vi "mtg reader - get short file names.vi"(6 "rowsize":i32=6, 9 "session file selection":refnum<vi>, 10 "session files in":refnum<vi>, 11 "data (session)":path) -> (2 "session files out":refnum<vi>)   [LabVIEW 2025]
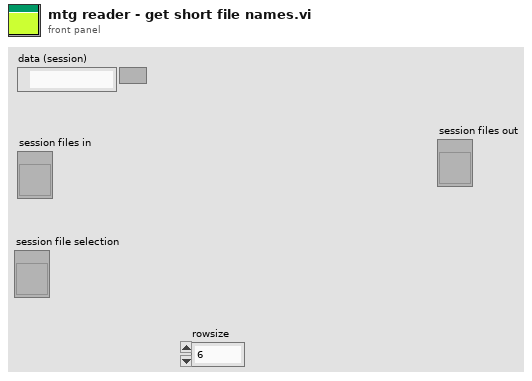
[diagram p1: front panel]
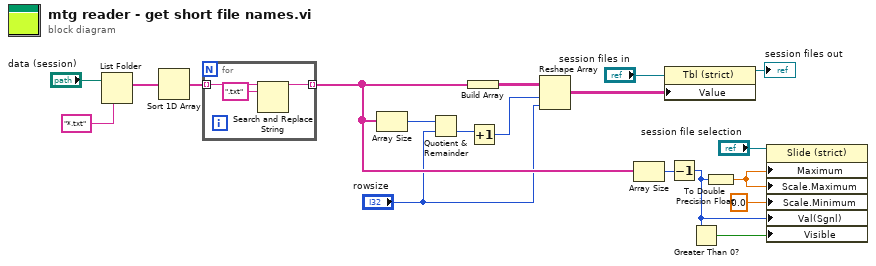
[diagram p0: block diagram]
diagram:
  n1 = List Folder(path="data (session)", pattern="*.txt") -> (filenames=w17:string[])  [unwired: 2 in, 3 out]
  n2 = Sort 1D Array(array=w17) -> (sorted array=w19:string[])
  n3 = for {
    tunnel: w19 -> [w22] mode=indexing
    tunnel: [w20] -> w6 mode=indexing
    n4 = Search and Replace String(input string=w22, search string=".txt") -> (result string=w20:string)  [unwired: 6 in, 3 out]
  }
  n5 = Array Size(array=w6) -> (size(s)=w14:i32)
  n6 = Quotient & Remainder(x=w14, y="rowsize") -> (floor(x/y)=w13:i32)  [unwired: 1 out]
  n7 = Build Array(w6) -> (w15:string[][])
  n8 = Increment(x=w13) -> (x+1=w12:i32)
  n9 = Reshape Array(w15, w12, "rowsize") -> (w8:string[][])
  n10 = Array Size(array=w6) -> (size(s)=w9:i32)
  n11 = property class="Tbl (strict)"(reference="session files in", "Value"=w8) -> (reference out=→"session files out":refnum<vi>)  [unwired: 1 in, 1 out]
  n12 = Decrement(x=w9) -> (x-1=w3:i32)
  n13 = Greater Than 0?(x=w3) -> (x > 0?=w4:bool)
  n14 = To Double Precision Float(number=w3) -> (double precision float=w2:dbl)
  n15 = property class="Slide (strict)"(reference="session file selection", "Maximum"=w2, "Scale.Maximum"=w2, "Scale.Minimum"=0.0 ("Scale.Range:Minimum"), "Val(Sgnl)"=w3, "Visible"=w4) -> ()  [unwired: 1 in, 2 out]
